vi "get default name.vi"(8 "error in":errorcluster, 11 "Targets in":refnum<class "Targets.lvclass">) -> (0 "error out":errorcluster, 2 "default name":string, 3 "Targets out":refnum<class "Targets.lvclass">)   [LabVIEW 2013, in "PL Framework Configuration Tool.lvlib" / "Targets.lvclass"]
uses:
  Targets.lvclass
  Framework Configuration Classes/target configuration/PL_Target Configuration.lvclass
  Framework Configuration Classes/target configuration/PL_Target Configuration.lvclass/PL_Target Configuration.ctl
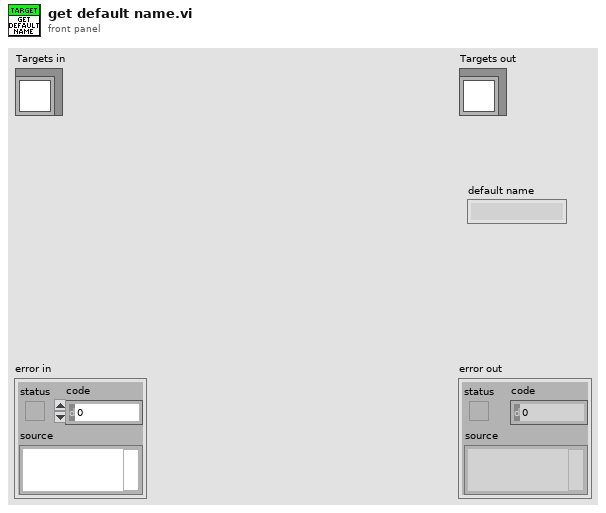
[diagram p1: front panel]
types:
  T1 = typedef "TBM configuration.lvclass/Target Types.ctl" = enum16{"Windows", "Mac", "Linux", "Linux RT ARM", "VxWorks", "Pharlap", "Other", "Linux RT x64"}
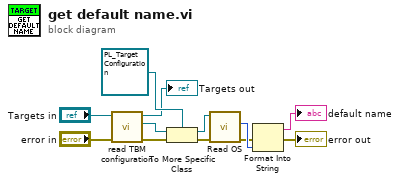
[diagram p0: block diagram]
diagram:
  n1 = call-dynamic "read TBM configuration.vi"("error in"="error in", "TBM Configuration Node in"="Targets in") -> ("error out"=w6:errorcluster, "configuration"=w7:refnum<class "TBM configuration.lvclass">, "TBM Configuration Node out"=→"Targets out":refnum<class "Targets.lvclass">)  [unwired: 7 in]
  n2 = To More Specific Class(target class=refnum<class "PL_Target Configuration.lvclass"> refnum ("Target Configuration"), reference=w7, error in=w6) -> (specific class reference=w3:refnum<class "PL_Target Configuration.lvclass">, error out=w4:errorcluster)
  n3 = call "Read OS.vi"("error in"=w4, "PL_Target Configuration in"=w3) -> ("error out"=w1:errorcluster, "Target Types"=w2:T1)  [unwired: 7 in, 1 out]
  n4 = Format Into String(error in=w1, w2) -> (resulting string=→"default name":string, error out=→"error out":errorcluster)  [unwired: 2 in]
